vi "String Compare Sequence.vi"() -> (2 "Sequence":refnum<class "Sequence Config.lvclass">)   [LabVIEW 2015, in "Sequencer Module tests.lvlib"]
uses:
  Sequencer Module tests.lvlib
  classes/Sequence/Config/Sequence Config.lvclass
  basic steps/String Compare/Config/String Compare Config.lvclass
  <vilib>/NI/Tag Bus/tag/Data Type.ctl
  <vilib>/NI/Tag Bus Module Framework/channel/channel classification.ctl
  basic steps/String Compare/Config/Mode.ctl
  basic steps/String Compare/Config/String Compare Config.lvclass/String Compare Config.ctl
  basic steps/String Compare/Config/Write Test Value Channel.vi
  basic steps/String Compare/Config/Write Result Channel.vi
  basic steps/String Compare/Config/Write Mode.vi
  basic steps/String Compare/Config/Write Limit_Regex.vi
  basic steps/String Compare/Config/Write ignore case.vi
  basic steps/String Compare/Config/Write Multiline.vi
  basic steps/String Compare/Config/Write offset.vi
  <vilib>/NI/Tag Bus/tag/tag descriptor.lvclass
  <vilib>/NI/Tag Bus Module Framework/channel/TBM channel.lvclass
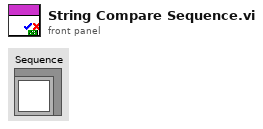
[diagram p1: front panel]
types:
  T1 = typedef "String Compare Config.lvclass/Mode.ctl" = enum16{"Compare Strings", "Match Regex"}
  T2 = typedef "TBM channel.lvclass/channel classification.ctl" = enum16{"input data", "output data", "processing parameter", "processing result"}
  T3 = typedef "tag bus.lvlib/tag descriptor.lvclass/Data Type.ctl" = enum16{"Double", "Single", "I64", "I32", "I16", "I8", "U64", "U32", "U16", "U8", "Boolean", "String", "Array of Double", "Array of Single", "Array of I64", "Array of I32", "Array of I16", "Array of I8", "Array of U64", "Array of U32", "Array of U16", "Array of U8", "Array of Boolean", "Array of String"}
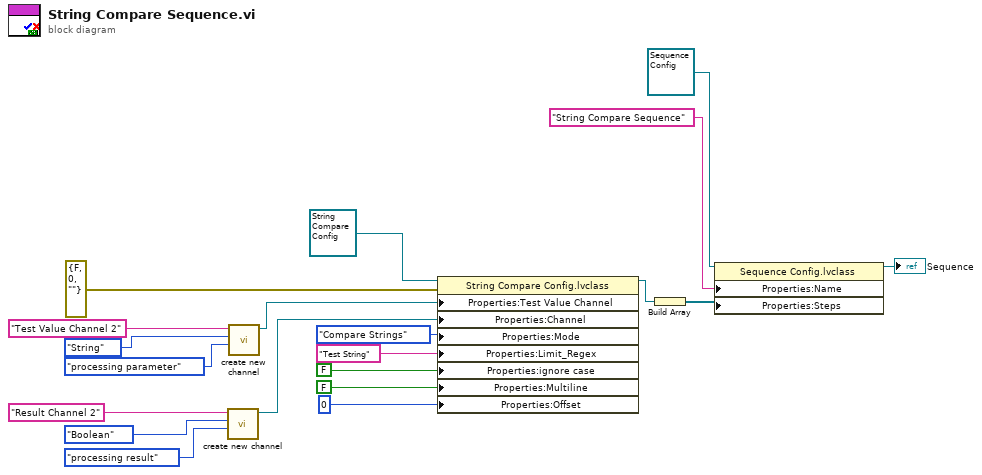
[diagram p0: block diagram]
diagram:
  n1 = call <vilib>:"create new channel.vi"("channel classification"=channel_classification."processing result", "data type"=Data_Type."Boolean", "channel name"="Result Channel 2") -> ("channel"=w9:refnum<class "TBM channel.lvclass">)  [unwired: 8 in]
  n2 = call <vilib>:"create new channel.vi"("channel classification"=channel_classification."processing parameter", "data type"=Data_Type."String" ("Data Type"), "channel name"="Test Value Channel 2" ("Jump Tag Name")) -> ("channel"=w13:refnum<class "TBM channel.lvclass">)  [unwired: 8 in]
  n3 = property class="String Compare Config.lvclass"(reference=refnum<class "String Compare Config.lvclass"> refnum ("String Compare Config.lvclass"), error in=errorcluster {"status"=FALSE, "code"=0, "source"=""} ("error in (no error)"), "Properties:Test Value Channel"=w13, "Properties:Channel"=w9, "Properties:Mode"=Mode."Compare Strings" ("Mode"), "Properties:Limit_Regex"="Test String" ("Limit_Regex"), "Properties:ignore case"=FALSE ("ignore case"), "Properties:Multiline"=FALSE ("Multiline"), "Properties:Offset"=0 ("Offset")) -> (reference out=w2:refnum<class "String Compare Config.lvclass">)  [unwired: 1 out]
  n4 = Build Array(w2) -> (w18:refnum<class "String Compare Config.lvclass">[])
  n5 = property class="Sequence Config.lvclass"(reference=refnum<class "Sequence Config.lvclass"> refnum ("Sequence Config.lvclass"), "Properties:Name"="String Compare Sequence" ("Name"), "Properties:Steps"=w18) -> (reference out=→"Sequence":refnum<class "Sequence Config.lvclass">)  [unwired: 1 in, 1 out]
